vi "Configure Triggered Source Measurement.vi"(0 "SMU Handle in":refnum<k15>, 1 "Active Channel":string, 5 "SMU Measurement Settings":T1={"DC Trigger Type"=enum."Immediate", "Measurement Trigger Input"="PXI_Trig0", "Measurement Time (s)"=0.001, "Measurement Mode"=enum."Single Point"} {"Measurement Time (s)" format="%#_13p"}, 11 "error in (no error)":errorcluster) -> (4 "SMU Handle out":refnum<k15>, 15 "error out":errorcluster)   [LabVIEW 2016, in "SMU.lvlib"]
uses:
  SMU.lvlib
  Typedefs/Supply Line Measurement Settings.ctl
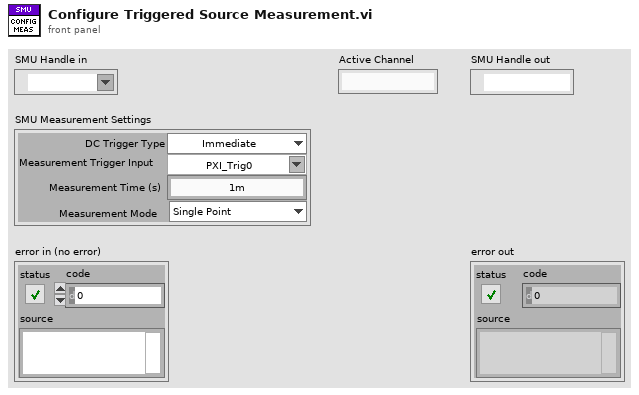
[diagram p1: front panel]
types:
  T1 = typedef "SMU.lvlib/Supply Line Measurement Settings.ctl" = cluster{"DC Trigger Type":enum16{"Immediate", "Digital Edge"}, "Measurement Trigger Input":string, "Measurement Time (s)":dbl, "Measurement Mode":enum16{"Single Point", "Record"}}
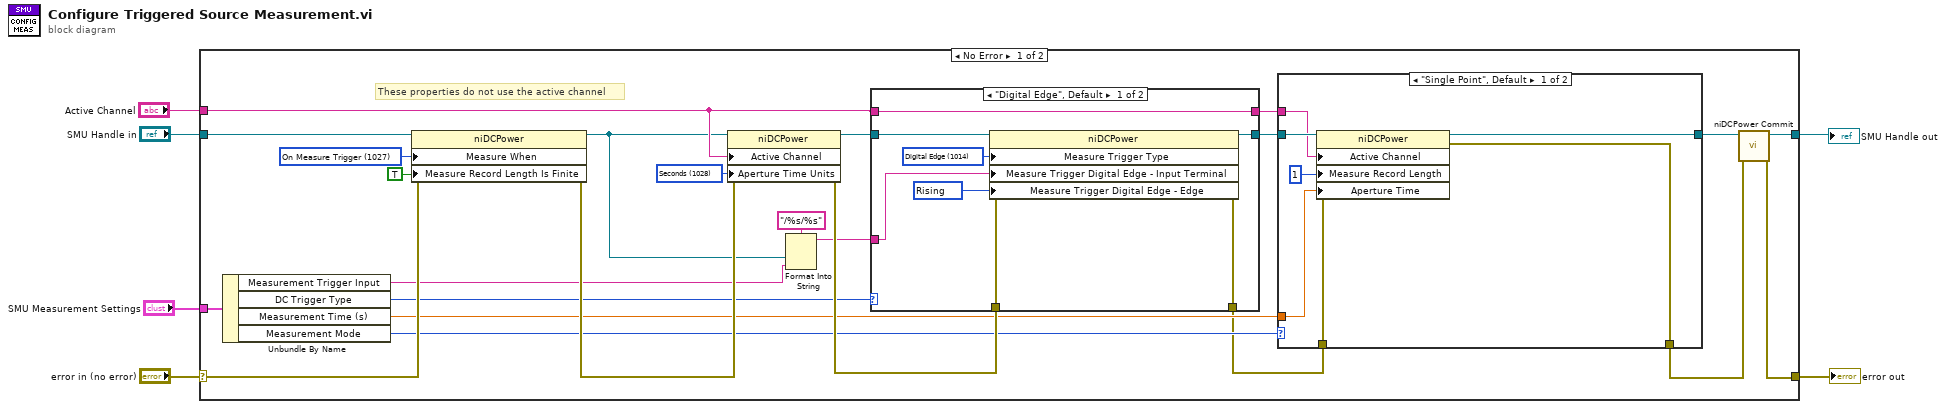
[diagram p0: block diagram]
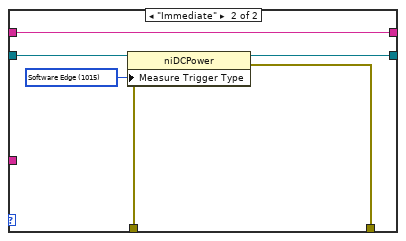
[diagram p2: hidden frame]
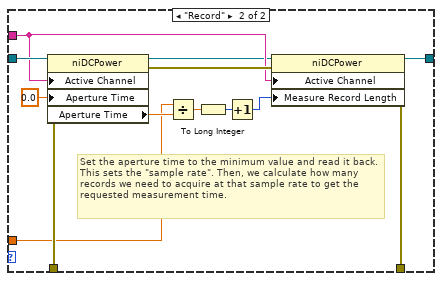
[diagram p3: hidden frame]
diagram:
  n1 = case shown="No Error" "error in (no error)" {
    selector: "error in (no error)" -> [w29 w66]
    tunnel: [w7 w66] -> w5
    tunnel: [w9 w65] -> w4
    tunnel: "SMU Handle in" -> [w22 w65]
    tunnel: "SMU Measurement Settings" -> [w24 _]
    tunnel: "Active Channel" -> [w19 _]
    frame No Error {
      w14 = 1027 items=["Automatically after Source Complete"=1025, "On Demand"=1026, "On Measure Trigger"=1027] ("Measurement:Advanced:Measure When")
      w12 = 1028 items=["Seconds"=1028, "Power Line Cycles"=1029] ("Measurement:Aperture Time Units")
      # "These properties do not use the active channel"
      n2 = Unbundle By Name(w24) -> ("Measurement Trigger Input"=w23:string, "DC Trigger Type"=w21:enum16{"Immediate", "Digital Edge"}, "Measurement Time (s)"=w16:dbl, "Measurement Mode"=w17:enum16{"Single Point", "Record"})
      n3 = property class="niDCPower"(reference=w22, error in=w29, "Measure When"=w14, "Measure Record Length Is Finite"=TRUE ("Measurement:Measure Record Length Is Finite")) -> (reference out=w15:refnum<k15>, error out=w28:errorcluster)
      n4 = property class="niDCPower"(reference=w15, error in=w28, "Active Channel"=w19, "Aperture Time Units"=w12) -> (reference out=w26:refnum<k15>, error out=w30:errorcluster)
      n5 = Format Into String(format string="/%s/%s", w15, w23) -> (resulting string=w25:string)  [unwired: 2 in, 1 out]
      n6 = case shown="\"Digital Edge\", Default" w21 {
        tunnel: w26 -> [w36 w42]
        tunnel: w30 -> [w38 w44]
        tunnel: [w37 w43] -> w10
        tunnel: [w35 w41] -> w11
        tunnel: w25 -> [w34 _]
        tunnel: w19 -> [w31 w39]
        tunnel: [w31 w39] -> w18
        frame "Digital Edge", Default {
          w32 = 1016 items=["Rising"=1016, "Falling"=1017] ("Triggers:Measure Trigger:Digital Edge:Edge")
          w33 = 1014 items=["Digital Edge"=1014, "Software Edge"=1015, "None"=1012] ("Triggers:Measure Trigger:Trigger Type")
          n7 = property class="niDCPower"(reference=w36, error in=w38, "Measure Trigger Type"=w33, "Measure Trigger Digital Edge - Input Terminal"=w34, "Measure Trigger Digital Edge - Edge"=w32) -> (reference out=w35:refnum<k15>, error out=w37:errorcluster)
        }
        frame "Immediate" {
          w40 = 1015 items=["Digital Edge"=1014, "Software Edge"=1015, "None"=1012] ("Triggers:Measure Trigger:Trigger Type")
          n8 = property class="niDCPower"(reference=w42, error in=w44, "Measure Trigger Type"=w40) -> (reference out=w41:refnum<k15>, error out=w43:errorcluster)
        }
      }
      n9 = case shown="\"Single Point\", Default" w17 {
        tunnel: w10 -> [w51 w64]
        tunnel: w11 -> [w49 w61]
        tunnel: [w50 w63] -> w8
        tunnel: [w48 w60] -> w20
        tunnel: w18 -> [w45 w59]
        tunnel: w16 -> [w46 w52]
        frame "Single Point", Default {
          n10 = property class="niDCPower"(reference=w49, error in=w51, "Active Channel"=w45, "Measure Record Length"=1 ("Measurement:Measure Record Length"), "Aperture Time"=w46) -> (reference out=w48:refnum<k15>, error out=w50:errorcluster)
        }
        frame "Record" {
          # "Set the aperture time to the minimum value and read it back. This sets the \"sample rate\". Then, we calculate how many records we need to acquire at that sample rate to get the requested measurement time."
          n11 = property class="niDCPower"(reference=w61, error in=w64, "Active Channel"=w59, "Aperture Time"=0.0 ("Measurement:Aperture Time")) -> (reference out=w57:refnum<k15>, error out=w62:errorcluster, "Aperture Time"=w58:dbl)
          n12 = Divide(x=w52, y=w58) -> (x/y=w56:dbl)
          n13 = To Long Integer(number=w56) -> (32bit integer=w55:i32)
          n14 = Increment(x=w55) -> (x+1=w54:i32)
          n15 = property class="niDCPower"(reference=w57, error in=w62, "Active Channel"=w59, "Measure Record Length"=w54) -> (reference out=w60:refnum<k15>, error out=w63:errorcluster)
        }
      }
      n16 = call <instrlib>:"niDCPower Commit.vi"("error in (no error)"=w8, "instrument handle"=w20) -> ("error out"=w7:errorcluster, "instrument handle out"=w9:refnum<k15>)  [unwired: 8 in]
    }
    frame Error {
    }
  }
  "SMU Handle out" <- w4
  "error out" <- w5
